vi "Tarea3_TaladroP2.vi"() -> ()   [LabVIEW 2025]
panel:
  out "Grande":dbl
  out "Chico":dbl
  in  "Encendido":bool
  out "Estado inicial":bool
  out "a 3":bool
  out "a2":bool
  in  "Apagado":bool
  out "a1":bool
  in  "Medida de la pieza":dbl=2.0 min=2.0 max=3.0 step=1.0
  # "INSTITUTO POLITÉCNICO NACIONAL\nUnidad Profesional Interdisciplinaria de Ingeniería \nCampus Zacatecas\n\nDe la Cruz García Yadira Arely\nGoytia Martínez Manuel"
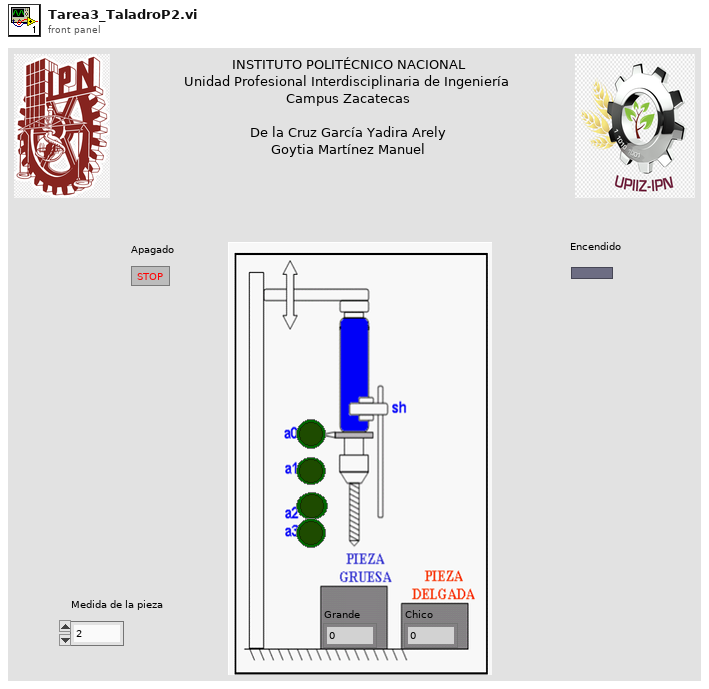
[diagram p1: front panel]
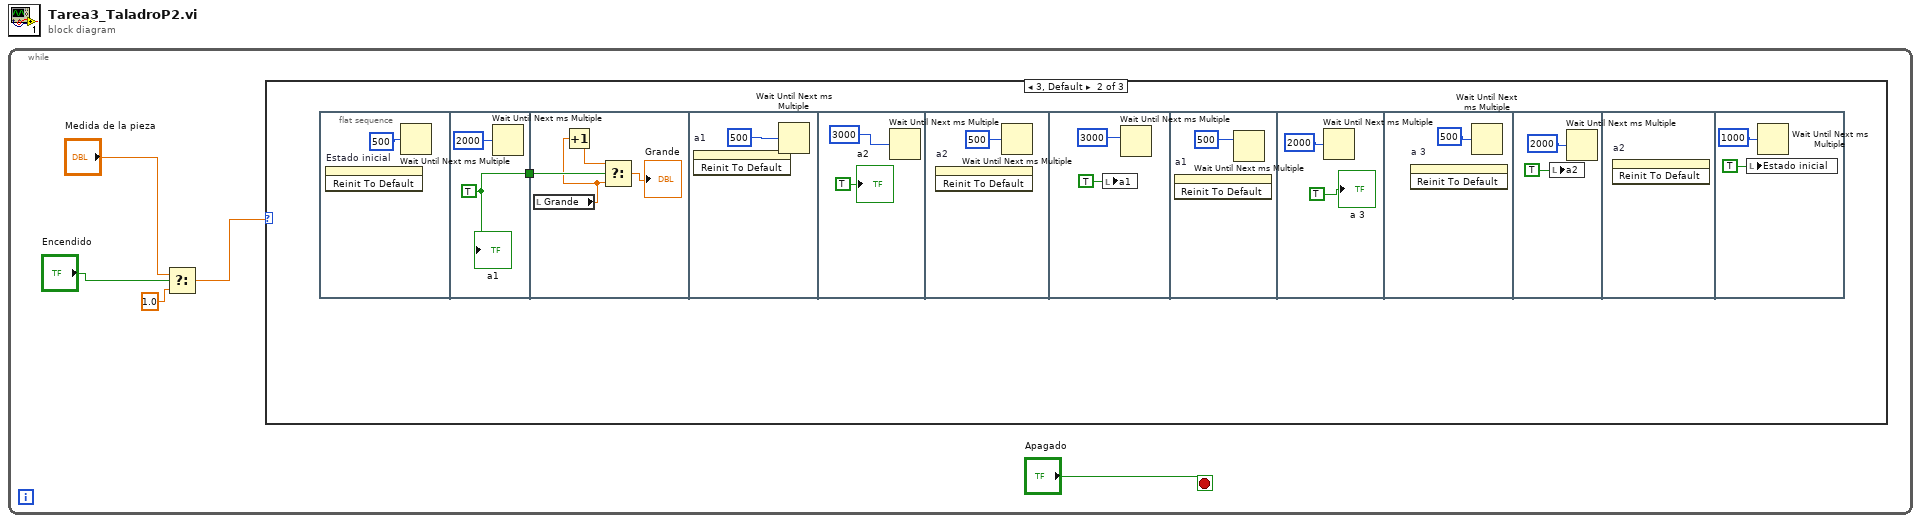
[diagram p0: block diagram]
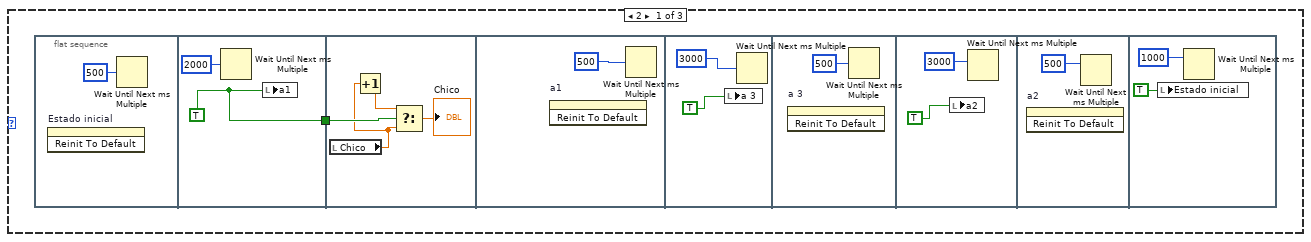
[diagram p2: hidden frame]
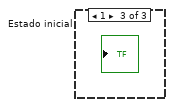
[diagram p3: hidden frame]
diagram:
  n1 = while {
    stop <- "Apagado" stop-if-true
    n2 = Select(t="Medida de la pieza", s="Encendido", f=1.0) -> (s? t:f=w4:dbl)
    n3 = case shown="3, Default" w4 {
      frame 2 {
        n4 = flat-sequence {
          tunnel: [w8] -> w6
          tunnel: w6 -> [w12]
          frame #0 {
            n5 = invoke on="Estado inicial" class="Bool (strict)" method="Reinit To Default"() -> ()  [unwired: 3 in, 3 out]
            n6 = Wait Until Next ms Multiple(millisecond multiple=u32 500) -> ()  [unwired: 1 out]
          }
          frame #1 {
            w8 = TRUE ("a1")
            n7 = Wait Until Next ms Multiple(millisecond multiple=u32 2000) -> ()  [unwired: 1 out]
            n8 = local write "a1"(w8) -> ()
          }
          frame #2 {
            n9 = local read "Chico"() -> (w10:dbl)
            n10 = Increment(x=w10) -> (x+1=w11:dbl)
            n11 = Select(t=w11, s=w12, f=w10) -> (s? t:f=→"Chico":dbl)
          }
          frame #3 {
            n12 = invoke on="a1" class="Bool (strict)" method="Reinit To Default"() -> ()  [unwired: 3 in, 3 out]
            n13 = Wait Until Next ms Multiple(millisecond multiple=u32 500) -> ()  [unwired: 1 out]
          }
          frame #4 {
            n14 = local write "a 3"(TRUE ("a 2")) -> ()
            n15 = Wait Until Next ms Multiple(millisecond multiple=u32 3000) -> ()  [unwired: 1 out]
          }
          frame #5 {
            n16 = invoke on="a 3" class="Bool (strict)" method="Reinit To Default"() -> ()  [unwired: 3 in, 3 out]
            n17 = Wait Until Next ms Multiple(millisecond multiple=u32 500) -> ()  [unwired: 1 out]
          }
          frame #6 {
            n18 = local write "a2"(TRUE ("a1")) -> ()
            n19 = Wait Until Next ms Multiple(millisecond multiple=u32 3000) -> ()  [unwired: 1 out]
          }
          frame #7 {
            n20 = invoke on="a2" class="Bool (strict)" method="Reinit To Default"() -> ()  [unwired: 3 in, 3 out]
            n21 = Wait Until Next ms Multiple(millisecond multiple=u32 500) -> ()  [unwired: 1 out]
          }
          frame #8 {
            n22 = local write "Estado inicial"(TRUE ("Estado inicial")) -> ()
            n23 = Wait Until Next ms Multiple(millisecond multiple=u32 1000) -> ()  [unwired: 1 out]
          }
        }
      }
      frame 3, Default {
        n24 = flat-sequence {
          tunnel: [w25] -> w23
          tunnel: w23 -> [w28]
          frame #0 {
            n25 = invoke on="Estado inicial" class="Bool (strict)" method="Reinit To Default"() -> ()  [unwired: 3 in, 3 out]
            n26 = Wait Until Next ms Multiple(millisecond multiple=u32 500) -> ()  [unwired: 1 out]
          }
          frame #1 {
            w25 = TRUE ("a1")
            n27 = Wait Until Next ms Multiple(millisecond multiple=u32 2000) -> ()  [unwired: 1 out]
            "a1" <- w25
          }
          frame #2 {
            n28 = local read "Grande"() -> (w27:dbl)
            n29 = Increment(x=w27) -> (x+1=w30:dbl)
            n30 = Select(t=w30, s=w28, f=w27) -> (s? t:f=→"Grande":dbl)
          }
          frame #3 {
            n31 = invoke on="a1" class="Bool (strict)" method="Reinit To Default"() -> ()  [unwired: 3 in, 3 out]
            n32 = Wait Until Next ms Multiple(millisecond multiple=u32 500) -> ()  [unwired: 1 out]
          }
          frame #4 {
            n33 = Wait Until Next ms Multiple(millisecond multiple=u32 3000) -> ()  [unwired: 1 out]
            "a2" <- TRUE ("a 2")
          }
          frame #5 {
            n34 = invoke on="a2" class="Bool (strict)" method="Reinit To Default"() -> ()  [unwired: 3 in, 3 out]
            n35 = Wait Until Next ms Multiple(millisecond multiple=u32 500) -> ()  [unwired: 1 out]
          }
          frame #6 {
            n36 = local write "a1"(TRUE ("a1")) -> ()
            n37 = Wait Until Next ms Multiple(millisecond multiple=u32 3000) -> ()  [unwired: 1 out]
          }
          frame #7 {
            n38 = invoke on="a1" class="Bool (strict)" method="Reinit To Default"() -> ()  [unwired: 3 in, 3 out]
            n39 = Wait Until Next ms Multiple(millisecond multiple=u32 500) -> ()  [unwired: 1 out]
          }
          frame #8 {
            n40 = Wait Until Next ms Multiple(millisecond multiple=u32 2000) -> ()  [unwired: 1 out]
            "a 3" <- TRUE ("a 3")
          }
          frame #9 {
            n41 = invoke on="a 3" class="Bool (strict)" method="Reinit To Default"() -> ()  [unwired: 3 in, 3 out]
            n42 = Wait Until Next ms Multiple(millisecond multiple=u32 500) -> ()  [unwired: 1 out]
          }
          frame #10 {
            n43 = local write "a2"(TRUE ("a 2")) -> ()
            n44 = Wait Until Next ms Multiple(millisecond multiple=u32 2000) -> ()  [unwired: 1 out]
          }
          frame #11 {
            n45 = invoke on="a2" class="Bool (strict)" method="Reinit To Default"() -> ()  [unwired: 3 in, 3 out]
          }
          frame #12 {
            n46 = local write "Estado inicial"(TRUE ("Estado inicial")) -> ()
            n47 = Wait Until Next ms Multiple(millisecond multiple=u32 1000) -> ()  [unwired: 1 out]
          }
        }
      }
      frame 1 {
      }
    }
  }
